vi "Pad array with wrap around data (dbl).vi"(9 "Extra wrap around data (5%)":dbl=5.0 min=5.0 max=100.0, 11 "Data In":dbl[][](array[numeric])) -> (1 "Pad Size":i32, 2 "Original Size":i32, 3 "Padded Array":dbl[][](array[numeric]))   [LabVIEW 2013]
doc: "Wraps data by specified percent"
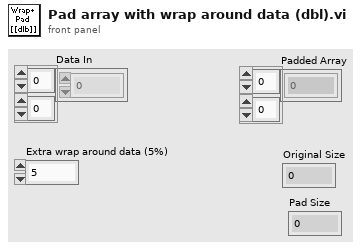
[diagram p1: front panel]
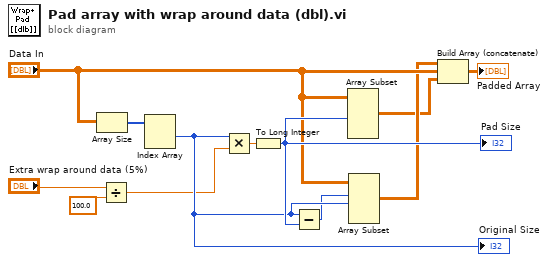
[diagram p0: block diagram]
diagram:
  n1 = Array Size(array="Data In") -> (size(s)=w1:i32[])
  n2 = Divide(x="Extra wrap around data (5%)", y=100.0) -> (x/y=w6:dbl)
  n3 = Index Array(array=w1) -> (element #1=w9:i32)  [unwired: 2 in, 1 out]
  "Original Size" <- w9
  n4 = Multiply(x=w9, y=w6) -> (x*y=w11:dbl)
  n5 = To Long Integer(number=w11) -> (32bit integer=w12:i32)
  "Pad Size" <- w12
  n6 = Subtract(x=w9, y=w12) -> (x-y=w2:i32)
  n7 = Array Subset(array="Data In", length (row)=w12) -> (w3:dbl[][])  [unwired: 3 in]
  n8 = Array Subset(array="Data In", index (row)=w2, length (row)=w9) -> (w7:dbl[][])  [unwired: 2 in]
  n9 = Build Array (concatenate)(w7, "Data In", w3) -> (→"Padded Array":dbl[][])
